vi "CreateLogMessage.vi"(11 "Command byte array":u32[](array[numeric])) -> (3 "Log Message":string)   [LabVIEW 2018]
doc: "Creates string message for a log file based on a command byte array."
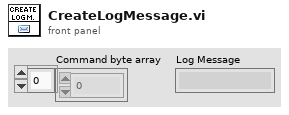
[diagram p1: front panel]
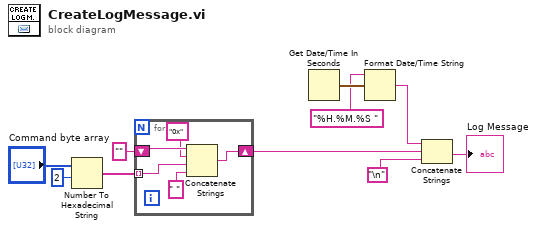
[diagram p0: block diagram]
diagram:
  n1 = Number To Hexadecimal String(1:i16 2 ("width (-)"), 2:"Command byte array") -> (0:w4:string[])
  n2 = for {
    shift-right: [w14] -> w7
    shift-left: "" -> [w15]
    tunnel: w4 -> [w13] mode=indexing
    n3 = Concatenate Strings(w15, "0x" ("string"), w13, " " ("string")) -> (w14:string)
  }
  n4 = Get Date/Time In Seconds() -> (seconds since 1Jan1904=w9:timestamp)
  n5 = Format Date/Time String(time format string (%c)="%H.%M.%S ", seconds (now)=w9) -> (date/time string=w10:string)  [unwired: 1 in]
  n6 = Concatenate Strings(w10, w7, "\n") -> (→"Log Message":string)
